vi "Encode (Multi-Message).vi"(7 "param map":T1, 11 "parameters in":dbl[](array[numeric])) -> (3 "words out":u16[](array[numeric]))   [LabVIEW 2020]
uses:
  RT Driver/RT Driver/Controls/Asynchronous - Parameter map_type.ctl
  _typedefs/parameter_config_type.ctl
  _typedefs/parameter_config_type_type.ctl
  _typedefs/parameter_config_encoding_type.ctl
  RT Driver/Ballard MIL-1553 Engine.lvlib
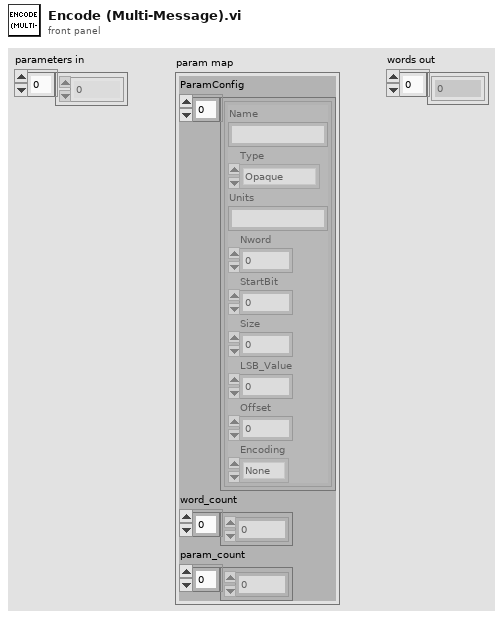
[diagram p1: front panel]
types:
  T1 = typedef "Ballard MIL-1553 Engine.lvlib/Asynchronous - Parameter map_type.ctl" = cluster{"ParamConfig":T2[], "word_count":u8[], "param_count":u8[]}
  T2 = typedef "parameter_config_type.ctl" = cluster{"Name":string, "Type":T3, "Units":string, "Nword":i32, "StartBit":i32, "Size":i32, "LSB_Value":i32, "Offset":i32, "Encoding":T4}
  T3 = typedef "parameter_config_type_type.ctl" = enum16{"Opaque", "Enum", "Float", "Integer", "Bcd", "Bool"}
  T4 = typedef "parameter_config_encoding_type.ctl" = enum16{"None", "2-complement", "Unsigned"}
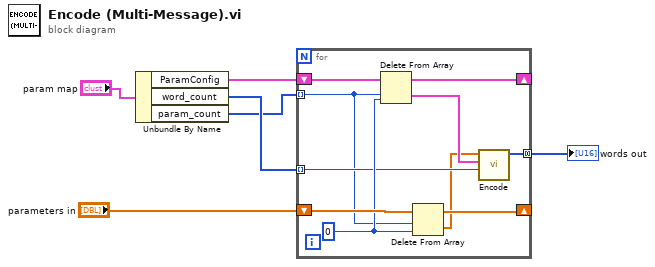
[diagram p0: block diagram]
diagram:
  n1 = Unbundle By Name("param map") -> ("ParamConfig"=w4:T2[], "word_count"=w5:u8[], "param_count"=w1:u8[])
  n2 = for {
    tunnel: w5 -> [w9] mode=indexing
    shift-right: [w15] -> _
    shift-left: w4 -> [w16]
    shift-right: [w12] -> _
    shift-left: "parameters in" -> [w14]
    tunnel: [w11] -> w2 mode=concatenating
    tunnel: w1 -> [w7] mode=indexing
    w13 = 0 ("index")
    n3 = Delete From Array(array=w16, length=w7, index=w13) -> (deleted portion=w10:T2[], array with subset deleted=w15:T2[])
    n4 = Delete From Array(array=w14, length=w7, index=w13) -> (deleted portion=w8:dbl[], array with subset deleted=w12:dbl[])
    n5 = call "Encode.vi"("word count"=w9, "param config"=w10, "parameters in"=w8) -> ("words out"=w11:u16[])  [unwired: 8 in]
  }
  "words out" <- w2
